vi "Dashboard Cursor Interpolation.vi"(5 "Remove Cursor":bool, 7 "Add Cursor":bool, 9 "Graph Detail":i32, 10 "Interpolation Method":i32(ring)=1 items=["nearest", "linear", "spline", "cubic Hermite", "Lagrange"], 11 "Interpolation Points":refnum<vi>) -> ()   [LabVIEW 2018]
uses:
  <vilib>/Utility/miscctls.llb/LVCursorListTypeDef.ctl
  <vilib>/gmath/NI_Gmath.lvlib
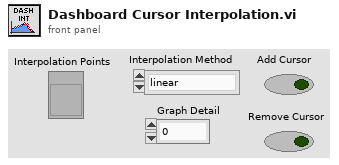
[diagram p1: front panel]
types:
  T1 = typedef "LVCursorListTypeDef.ctl" = cluster{"Name":string, "Color":u32, "Style":u8, "Point Style":u8, "Name Visible":bool, "Allow Drag":bool, "Cursor Mode":u32, "Plot":i32, "Index":i32, "Position":cluster{"X":dbl, "Y":dbl}, "X Scale":u32, "Y Scale":u32, "Watch Plots":i32[], "Watch All Plots":bool, "Plot Area":i32, "Label Offset":cluster{"X":dbl, "Y":dbl}}[]
  T2 = cluster{"Name":string, "Color":u32, "Style":u8, "Point Style":u8, "Name Visible":bool, "Allow Drag":bool, "Cursor Mode":u32, "Plot":i32, "Index":i32, "Position":cluster{"X":dbl, "Y":dbl}, "X Scale":u32, "Y Scale":u32, "Watch Plots":i32[], "Watch All Plots":bool, "Plot Area":i32, "Label Offset":cluster{"X":dbl, "Y":dbl}}
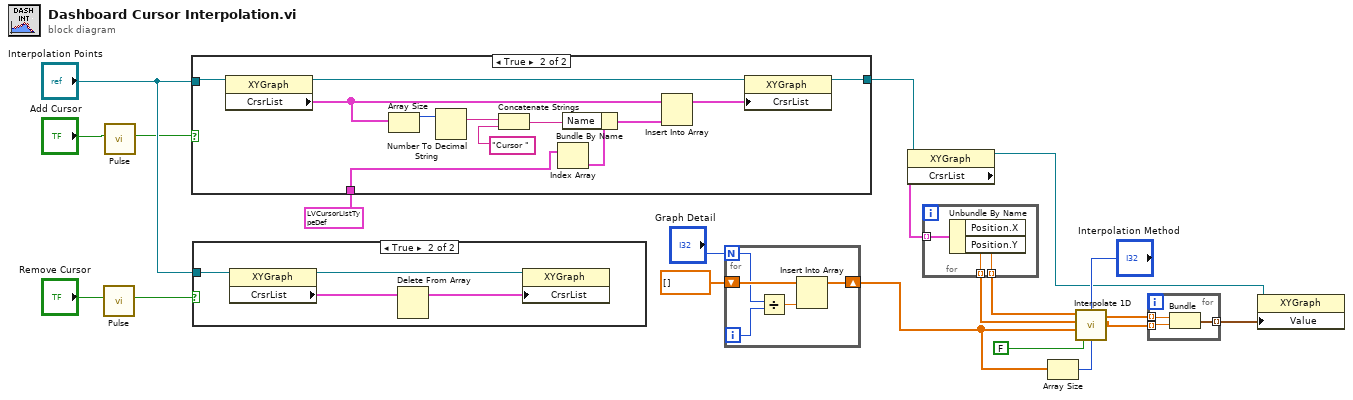
[diagram p0: block diagram]
diagram:
  n1 = call "Pulse.vi"("Input"="Remove Cursor") -> ("Output"=w3:bool)  [unwired: 10 in]
  n2 = call "Pulse.vi"("Input"="Add Cursor") -> ("Output"=w1:bool)  [unwired: 10 in]
  n3 = case shown="True" w1 {
    tunnel: T1 [{"Name"="Cursor 0", "Color"=33023, "Style"=0, "Point Style"=1, "Name Visible"=FALSE, "Allow Drag"=TRUE, "Cursor Mode"=0, "Plot"=0, "Index"=0, "Position"={"X"=0.5, "Y"=0.5}, "X Scale"=0, "Y Scale"=0, "Watch Plots"=[], "Watch All Plots"=FALSE, "Plot Area"=0, "Label Offset"={"X"=0.0, "Y"=0.0}}] ("Cursor List") -> [_ w30]
    tunnel: "Interpolation Points" -> [w21 w25]
    tunnel: [w21 w22] -> w6
    frame False {
    }
    frame True {
      n4 = property class="XYGraph"(reference=w25) -> (reference out=w24:refnum<vi>, "CrsrList"=w26:T1)  [unwired: 1 in, 1 out]
      n5 = Array Size(array=w26) -> (size(s)=w32:i32)
      n6 = Number To Decimal String(number=w32) -> (decimal integer string=w31:string)  [unwired: 1 in]
      n7 = Concatenate Strings("Cursor ", w31) -> (w28:string)
      n8 = Index Array(array=w30) -> (element=w29:T2)  [unwired: 1 in]
      n9 = Bundle By Name(cluster=w29, "Name"=w28) -> (w27:T2)
      n10 = Insert Into Array(array=w26, new element=w27) -> (w23:T1)  [unwired: 1 in]
      n11 = property class="XYGraph"(reference=w24, "CrsrList"=w23) -> (reference out=w22:refnum<vi>)  [unwired: 1 in, 1 out]
    }
  }
  n12 = case shown="True" w3 {
    tunnel: "Interpolation Points" -> [_ w35]
    frame False {
    }
    frame True {
      n13 = property class="XYGraph"(reference=w35) -> (reference out=w34:refnum<vi>, "CrsrList"=w36:T1)  [unwired: 1 in, 1 out]
      n14 = Delete From Array(array=w36) -> (array with subset deleted=w37:T1)  [unwired: 2 in, 1 out]
      n15 = property class="XYGraph"(reference=w34, "CrsrList"=w37) -> ()  [unwired: 1 in, 2 out]
    }
  }
  n16 = for {
    N: "Graph Detail" -> [w39]
    shift-right: [w41] -> w5
    shift-left: dbl[] [] -> [w40]
    i -> [w38]
    n17 = Divide(x=w38, y=w39) -> (x/y=w42:dbl)
    n18 = Insert Into Array(array=w40, new element=w42) -> (w41:dbl[])  [unwired: 1 in]
  }
  n19 = property class="XYGraph"(reference=w6) -> (reference out=w7:refnum<vi>, "CrsrList"=w11:T1)  [unwired: 1 in, 1 out]
  n20 = for {
    tunnel: w11 -> [w45] mode=indexing
    tunnel: [w44] -> w15 mode=indexing
    tunnel: [w43] -> w14 mode=indexing
    n21 = Unbundle By Name(w45) -> ("Position.X"=w44:dbl, "Position.Y"=w43:dbl)
  }
  n22 = Array Size(array=w5) -> (size(s)=w12:i32)
  n23 = call <vilib>:"Interpolate 1D.vi"("ntimes"=w12, "method"="Interpolation Method", "X is monotonic"=FALSE, "xi"=w5, "X"=w15, "Y"=w14) -> ("xi used"=w9:dbl[], "yi"=w10:dbl[])  [unwired: 3 in, 1 out]
  n24 = for {
    tunnel: w10 -> [w47] mode=indexing
    tunnel: w9 -> [w46] mode=indexing
    tunnel: [w48] -> w8 mode=indexing
    n25 = Bundle("Numeric"=w46, "Numeric"=w47) -> (w48:cluster{"Numeric":dbl, "Numeric":dbl})  [unwired: 1 in]
  }
  n26 = property class="XYGraph"(reference=w7, "Value"=w8) -> ()  [unwired: 1 in, 2 out]
